vi "Anritsu VNA Wait for Operation Complete (OPC).vi"(7 "Anritsu VNA":T1, 8 "error in (no error)":errorcluster, 9 "Timeout, ms (10000)":u32=10000, 11 "VISA Resource Name":refnum<visa-resource-name>) -> (0 "error out":errorcluster, 3 "dup VISA Resource Name":refnum<visa-resource-name>)   [LabVIEW 2011]
uses:
  TypeDefs/Anritsu VNA Instrument Info.ctl
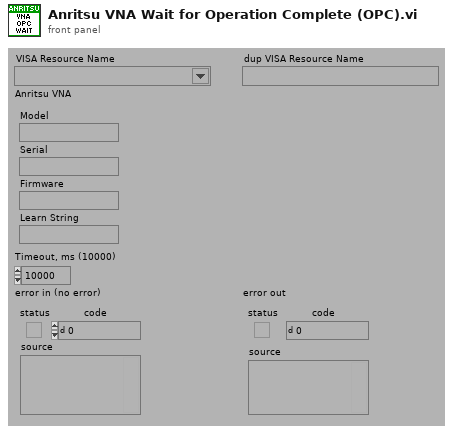
[diagram p1: front panel]
types:
  T1 = typedef "Anritsu VNA Instrument Info.ctl" = cluster{"Model":string, "Serial":string, "Firmware":string, "Learn String":string}
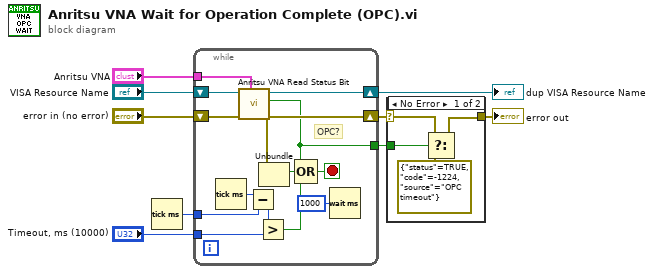
[diagram p0: block diagram]
diagram:
  n1 = Tick Count (ms)() -> (millisecond timer value=w9:u32)
  n2 = while {
    tunnel: [w10] -> w6
    tunnel: "Timeout, ms (10000)" -> [w20]
    tunnel: w9 -> [w23]
    shift-right: [w16] -> w5
    shift-left: "error in (no error)" -> [w17]
    shift-right: [w12] -> w2
    shift-left: "VISA Resource Name" -> [w18]
    tunnel: "Anritsu VNA" -> [w11]
    stop <- w13 stop-if-true
    # "OPC?"
    n3 = Tick Count (ms)() -> (millisecond timer value=w22:u32)
    n4 = call "Anritsu VNA Read Status Bit.vi"("Anritsu VNA"=w11, "error in (no error)"=w17, "VISA Resource Name"=w18) -> ("error out"=w16:errorcluster, "OPC Bit"=w10:bool, "dup VISA Resource Name"=w12:refnum<visa-resource-name>)  [unwired: 1 in, 5 out]
    n5 = Subtract(x=w22, y=w23) -> (x-y=w21:u32)
    n6 = Greater?(x=w21, y=w20) -> (0:w14:bool)
    n7 = Unbundle(w16) -> ("status"=w15:bool)  [unwired: 2 out]
    n8 = Compound Arithmetic op=OR(w10, w15, w14) -> (w13:bool)
    n9 = Wait (ms)(milliseconds to wait=u32 1000) -> ()  [unwired: 1 out]
  }
  "dup VISA Resource Name" <- w2
  n10 = case shown="No Error" w5 {
    selector: w5 -> [w26 w28]
    tunnel: w6 -> [w27 _]
    tunnel: [w25 w28] -> w4
    frame No Error {
      n11 = Select(t=w26, s=w27, f=errorcluster {"status"=TRUE, "code"=-1224, "source"="OPC timeout"}) -> (s? t:f=w25:errorcluster)
    }
    frame Error {
    }
  }
  "error out" <- w4
